vi "dadada.vi"() -> ()   [LabVIEW 2021]
uses:
  <vilib>/express/express analysis/Spectral/Block/exnSpectralBlock spectral measurements power poly.vi
  <vilib>/express/express analysis/Spectral/Block/exnSpectralBlock spectral measurements power DDT.vi
  <vilib>/express/express analysis/Spectral/XNode/ExpressSpectralMeasurementsBlockNode.xnode
panel:
  out "XY Graph 2":cluster{dbl[], "Y":dbl[]}(graph)
  out "XY Graph":cluster{dbl[], "Y":dbl[]}(graph)
  in  "rate":dbl=1000.0
  in  "number of samples":i32=100
  in  "stop":bool
  out "size(s) 3":i32
  out "dt 2":dbl
  out "Array":dbl[](array[numeric])
  out "size(s) 2":i32
  out "size(s)":i32
  out "Y 2":dbl[](array[numeric])
  out "Y":dbl[](array[numeric])
  out "dt":dbl
  out "Waveform":waveform(dbl)
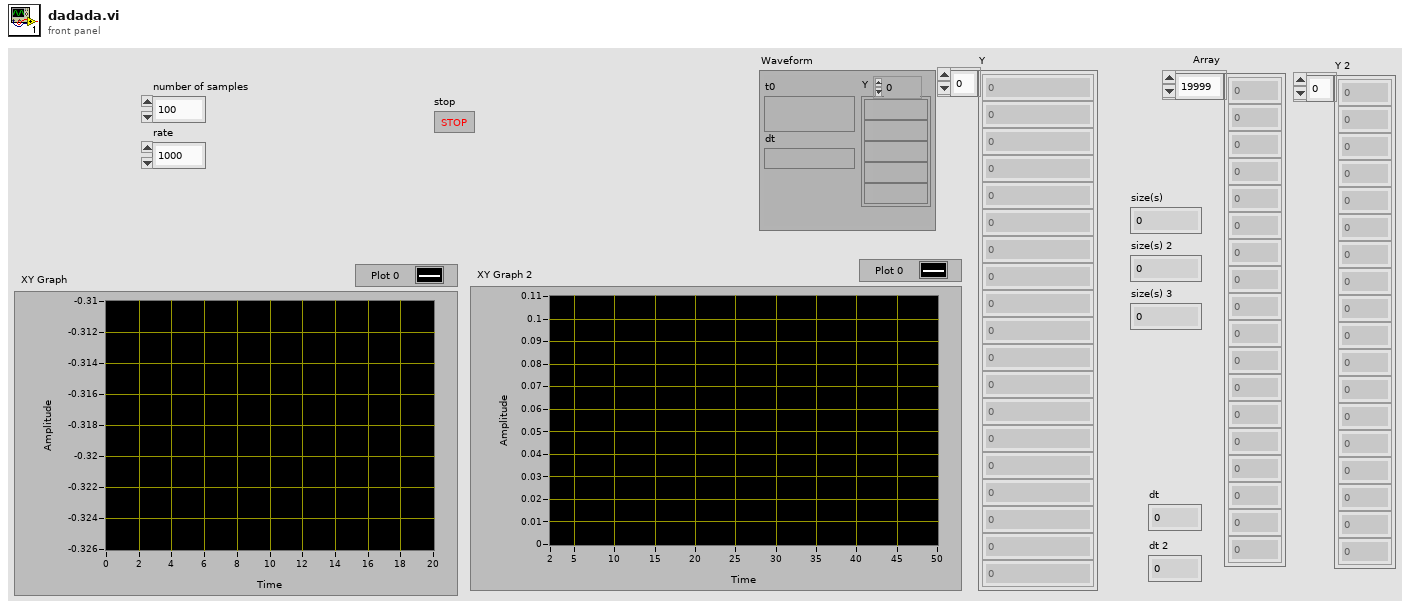
[diagram p1: front panel]
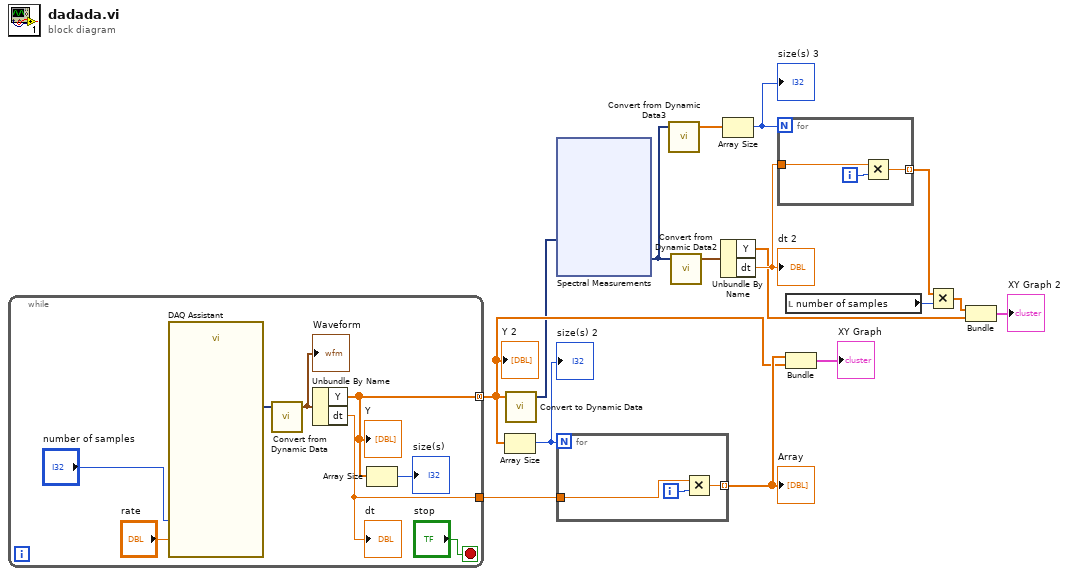
[diagram p0: block diagram]
diagram:
  n1 = while {
    tunnel: [w23] -> w12 mode=concatenating
    tunnel: [w21] -> w15
    stop <- "stop" stop-if-true
    n2 = call "DAQ Assistant"("rate"="rate", "number of samples"="number of samples") -> ("data"=w19:dynamicdata)  [unwired: 14 in, 3 out]
    n3 = call "Convert from Dynamic Data"("Dynamic Data Type"=w19) -> ("Waveform"=w24:waveform(dbl))  [unwired: 3 in]
    "Waveform" <- w24
    n4 = Unbundle By Name(w24) -> ("Y"=w23:dbl[], "dt"=w21:dbl)
    "dt" <- w21
    "Y" <- w23
    n5 = Array Size(array=w23) -> (size(s)=→"size(s)":i32)
  }
  "Y 2" <- w12
  n6 = Array Size(array=w12) -> (size(s)=w16:i32)
  "size(s) 2" <- w16
  n7 = call "Convert to Dynamic Data"("Array"=w12) -> ("Dynamic Data Type"=w11:dynamicdata)  [unwired: 3 in]
  n8 = xnode "Spectral Measurements"("Signals"=w11) -> ("Power Spectrum"=w10:dynamicdata)  [unwired: 1 in, 1 out]
  n9 = for {
    N: w16 -> [_]
    tunnel: w15 -> [w27]
    tunnel: [w25] -> w14 mode=indexing
    i -> [w26]
    n10 = Multiply(x=w27, y=w26) -> (x*y=w25:dbl)
  }
  "Array" <- w14
  n11 = call "Convert from Dynamic Data3"("Dynamic Data Type"=w10) -> ("Array"=w9:dbl[])  [unwired: 3 in]
  n12 = call "Convert from Dynamic Data2"("Dynamic Data Type"=w10) -> ("Waveform"=w13:waveform(dbl))  [unwired: 3 in]
  n13 = Unbundle By Name(w13) -> ("Y"=w7:dbl[], "dt"=w8:dbl)
  "dt 2" <- w8
  n14 = Array Size(array=w9) -> (size(s)=w6:i32)
  "size(s) 3" <- w6
  n15 = for {
    N: w6 -> [_]
    tunnel: w8 -> [w29]
    tunnel: [w28] -> w5 mode=indexing
    i -> [w30]
    n16 = Multiply(x=w29, y=w30) -> (x*y=w28:dbl)
  }
  n17 = local read "number of samples"() -> (w3:i32)
  n18 = Bundle(w14, "Y"=w12) -> (→"XY Graph":cluster{dbl[], "Y":dbl[]})  [unwired: 1 in]
  n19 = Multiply(x=w5, y=w3) -> (x*y=w4:dbl[])
  n20 = Bundle(w4, "Y"=w7) -> (→"XY Graph 2":cluster{dbl[], "Y":dbl[]})  [unwired: 1 in]
